vi "Check & Create Output Folders.vi"(8 "error in (no error)":errorcluster, 11 "Internal Data Cluster in":T1) -> (0 "error out":errorcluster, 3 "Internal Data Cluster out":T1)   [LabVIEW 2019, in "Package Builder.lvlib"]
uses:
  Package Builder.lvlib
  TypeDefs/Post-Build Action IDC.ctl
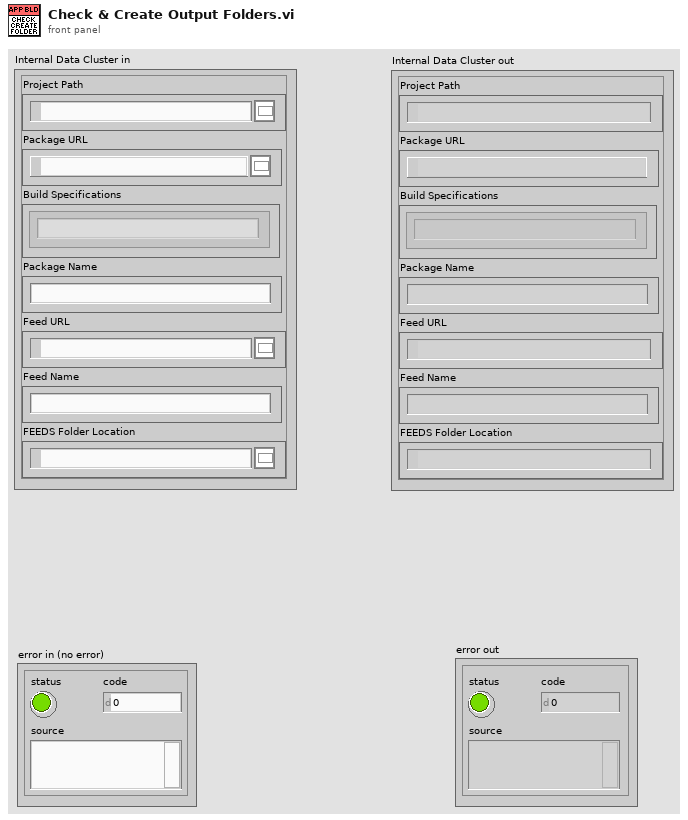
[diagram p1: front panel]
types:
  T1 = typedef "Package Builder.lvlib/Post-Build Action IDC.ctl" = cluster{"Project Path":path, "Package URL":path, "Build Specifications":string[], "Package Name":string, "Feed URL":path, "Feed Name":string, "FEEDS Folder Location":path}
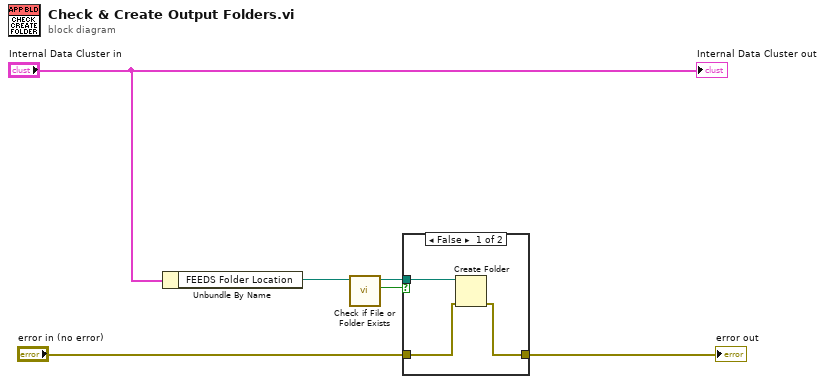
[diagram p0: block diagram]
diagram:
  n1 = Unbundle By Name("Internal Data Cluster in") -> ("FEEDS Folder Location"=w1:path)
  n2 = call <vilib>:"Check if File or Folder Exists.vi"("path"=w1) -> ("file or folder exists?"=w3:bool, "dup path"=w4:path)  [unwired: 8 in, 1 out]
  n3 = case shown="False" w3 {
    tunnel: w4 -> [w9 _]
    tunnel: "error in (no error)" -> [w8 w10]
    tunnel: [w7 w10] -> w6
    frame False {
      n4 = Create Folder(path (use dialog)=w9, error in=w8) -> (error out=w7:errorcluster)  [unwired: 1 in, 2 out]
    }
    frame True {
    }
  }
  "error out" <- w6
  "Internal Data Cluster out" <- "Internal Data Cluster in"
